vi "RSZVB Set Generator Attenuator Mode.vi"(7 "Attenuation Mode (0: Automatic)":i32(ring) items=["Automatic", "Manual", "Low Noise"], 8 "error in (no error)":errorcluster {"code" format="%.0x"}, 9 "Port (1)":i32=1, 10 "Channel (1)":i32=1, 11 "VISA session":refnum<visa-resource-name>) -> (0 "error out":errorcluster {"code" format="%.0x"}, 3 "dup VISA session":refnum<visa-resource-name>)   [LabVIEW 2011]
doc: "This VI defines how the attenuation factor for the generated wave at test port no. <Pt> is set. \n\nNote(s):\n\n(1) This VI can be used only with R&S ZVA and ZVB instruments.\n\nRemote-control command(s):\nSOURce<Ch>:POWer<Pt>:ATTenuation:MODE AUTO | MANual | LNOise"
uses:
  _utility/RSZVB Global Data.vi
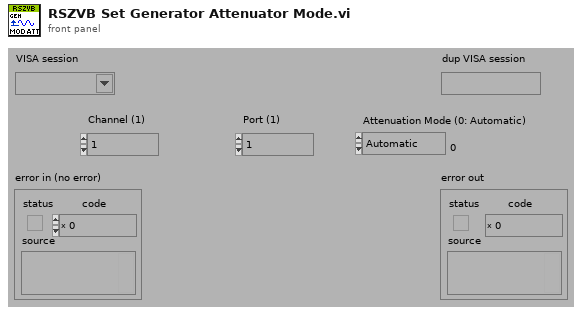
[diagram p1: front panel]
types:
  T1 = cluster{"Error Checking (T: On)":bool, "Installed Options":string[], "Data Valid?":bool, "Ports":i32, "Model":string[], "Option Checking (T: On)":bool}[]
  T2 = cluster{"Error Checking (T: On)":bool, "Installed Options":string[], "Data Valid?":bool, "Ports":i32, "Model":string[], "Option Checking (T: On)":bool}
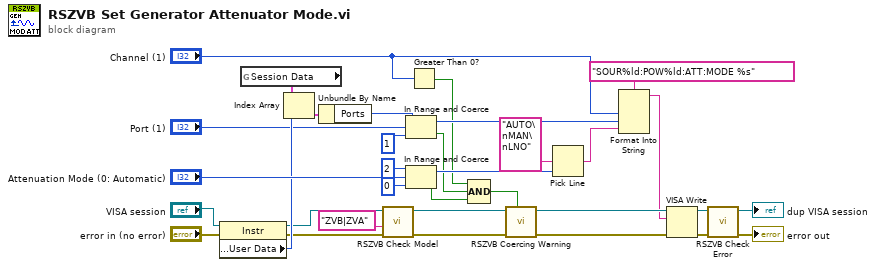
[diagram p0: block diagram]
diagram:
  n1 = property class="Instr"(reference="VISA session", error in="error in (no error)") -> (reference out=w15:refnum<visa-resource-name>, error out=w16:errorcluster, "General Settings:User Data"=w19:u32)
  n2 = global read "RSZVB Global Data.vi" "Session Data"() -> (w13:T1)
  n3 = Index Array(array=w13, index=w19) -> (element=w20:T2)
  n4 = Unbundle By Name(w20) -> ("Ports"=w14:i32)
  n5 = call "RSZVB Check Model.vi"("error in (no error)"=w16, "Model"="ZVB|ZVA" ("Options"), "VISA session"=w15) -> ("error out"=w27:errorcluster, "dup VISA session"=w26:refnum<visa-resource-name>)  [unwired: 7 in]
  n6 = In Range and Coerce(upper limit=w14, x="Port (1)", lower limit=1) -> (coerced(x)=w11:i32, In Range?=w5:bool)
  n7 = In Range and Coerce(upper limit=2, x="Attenuation Mode (0: Automatic)", lower limit=0) -> (coerced(x)=w22:i32, In Range?=w8:bool)
  n8 = Greater Than 0?(x="Channel (1)") -> (x > 0?=w4:bool)
  n9 = Compound Arithmetic op=AND(w4, w5, w8) -> (w3:bool)
  n10 = call "RSZVB Coercing Warning.vi"("In Range?"=w3, "error in (no error)"=w27, "VISA session"=w26) -> ("error out"=w31:errorcluster, "dup VISA session"=w32:refnum<visa-resource-name>)  [unwired: 7 in]
  n11 = Pick Line(multi-line string="AUTO\nMAN\nLNO", line index=w22) -> (output string=w1:string)  [unwired: 1 in]
  n12 = Format Into String(format string="SOUR%ld:POW%ld:ATT:MODE %s", "Channel (1)", w11, w1) -> (resulting string=w28:string)  [unwired: 2 in, 1 out]
  n13 = VISA Write(VISA resource name=w32, write buffer=w28, error in (no error)=w31) -> (VISA resource name out=w29:refnum<visa-resource-name>, error out=w30:errorcluster)  [unwired: 1 out]
  n14 = call "RSZVB Check Error.vi"("error in (no error)"=w30, "VISA session"=w29) -> ("error out"=→"error out":errorcluster, "dup VISA session"=→"dup VISA session":refnum<visa-resource-name>)  [unwired: 8 in]
